vi "Picture_shr_Save_to_matlab.vi"(8 "Input Cluster":T7, 9 "Stack":T1, 10 "Mode":enum32{"Confocal", "High Res"}(radio), 11 "Save":bool) -> ()   [LabVIEW 2009]
uses:
  atmcd32d.llb/AcquisitionMode_mode typedef.ctl
  atmcd32d.llb/ReadMode_mode typedef.ctl
  atmcd32d.llb/TriggerMode_mode typedef.ctl
  atmcd32d.llb/Shutter_type typedef.ctl
  atmcd32d.llb/Shutter_mode typedef.ctl
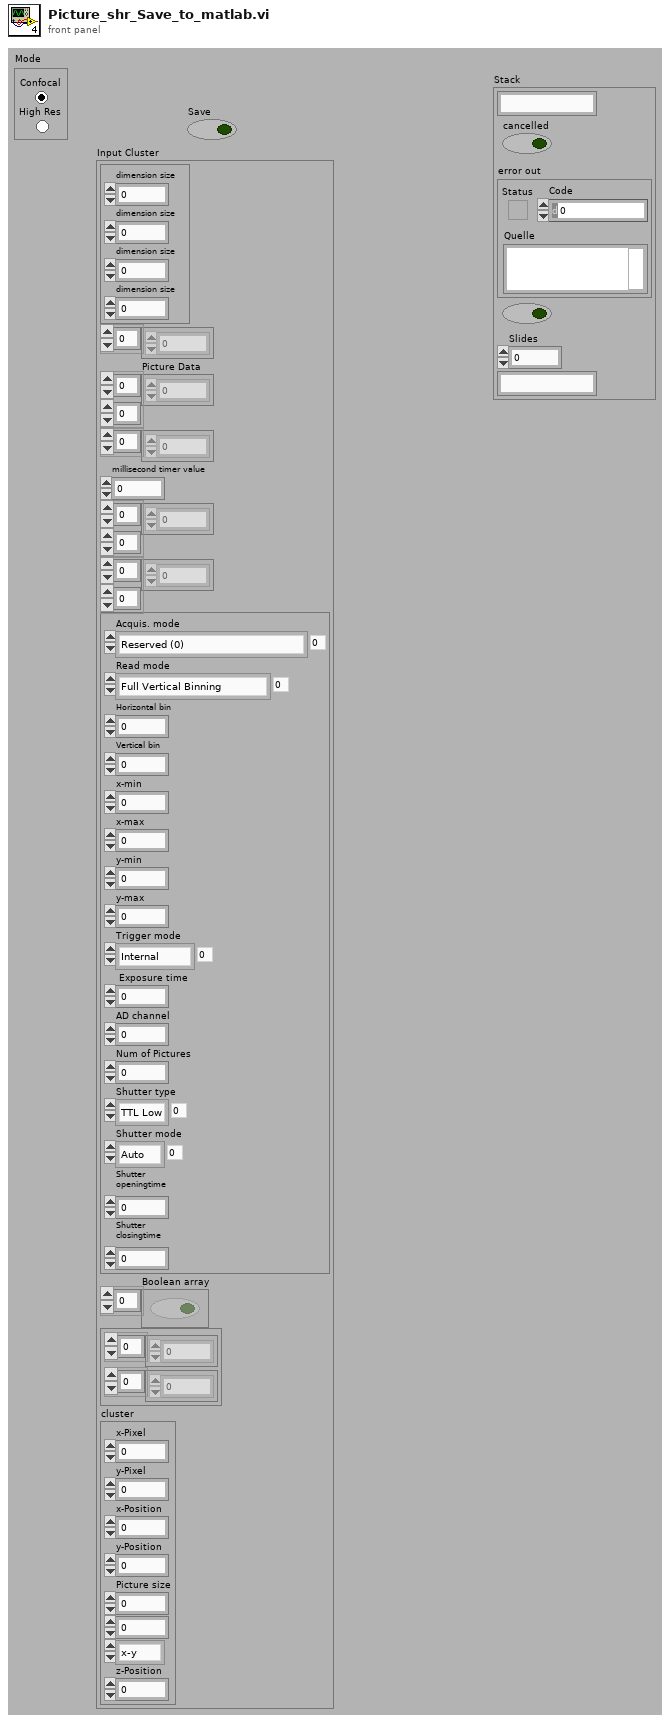
[diagram p1: front panel]
types:
  T1 = cluster{string, "cancelled":bool, "error out":errorcluster, bool, "Slides":i32, string}
  T2 = typedef "AcquisitionMode_mode typedef.ctl" = enum16{"Reserved (0)", "Single Scan", "Accumulate", "Kinetics", "Fast Kinetics", "Run Till Abort", "Reserved (6)", "Reserved (7)", "Reserved (8)", "Time Delayed Integration"}
  T3 = typedef "ReadMode_mode typedef.ctl" = enum16{"Full Vertical Binning", "Multi-Track", "Random-Track", "Single-Track", "Image"}
  T4 = typedef "TriggerMode_mode typedef.ctl" = enum16{"Internal", "External", "N/A (2)", "N/A (3)", "N/A (4)", "N/A (5)", "External Start"}
  T5 = typedef "Shutter_type typedef.ctl" = enum16{"TTL Low", "TTL High"}
  T6 = typedef "Shutter_mode typedef.ctl" = enum16{"Auto", "Open", "Close"}
  T7 = cluster{cluster{"dimension size":i32, "dimension size":i32, "dimension size":i32, "dimension size":i32}, i32[], "Picture Data":dbl[][], u32[], "millisecond timer value":u32, dbl[][], i32[][], cluster{"Acquis. mode":T2, "Read mode":T3, "Horizontal bin":i32, "Vertical bin":i32, "x-min":i32, "x-max":i32, "y-min":i32, "y-max":i32, "Trigger mode":T4, " Exposure time":sgl, "AD channel":i32, "Num of Pictures":i32, "Shutter type":T5, "Shutter mode":T6, "Shutter\nopeningtime":i32, "Shutter\nclosingtime":i32}, "Boolean array":bool[], cluster{dbl[], dbl[]}, "cluster":cluster{"x-Pixel":u16, "y-Pixel":u16, "x-Position":dbl, "y-Position":dbl, "Picture size":dbl, dbl, enum32{"x-y", "x-z", "y-z"}, "z-Position":dbl}}
  T8 = enum16{"open", "replace", "create", "open or create", "replace or create", "replace or create with confirmation"}
  T9 = cluster{"x-Pixel":u16, "y-Pixel":u16, "x-Position":dbl, "y-Position":dbl, "Picture size":dbl, dbl, enum32{"x-y", "x-z", "y-z"}, "z-Position":dbl}
  T10 = cluster{"Acquis. mode":T2, "Read mode":T3, "Horizontal bin":i32, "Vertical bin":i32, "x-min":i32, "x-max":i32, "y-min":i32, "y-max":i32, "Trigger mode":T4, " Exposure time":sgl, "AD channel":i32, "Num of Pictures":i32, "Shutter type":T5, "Shutter mode":T6, "Shutter\nopeningtime":i32, "Shutter\nclosingtime":i32}
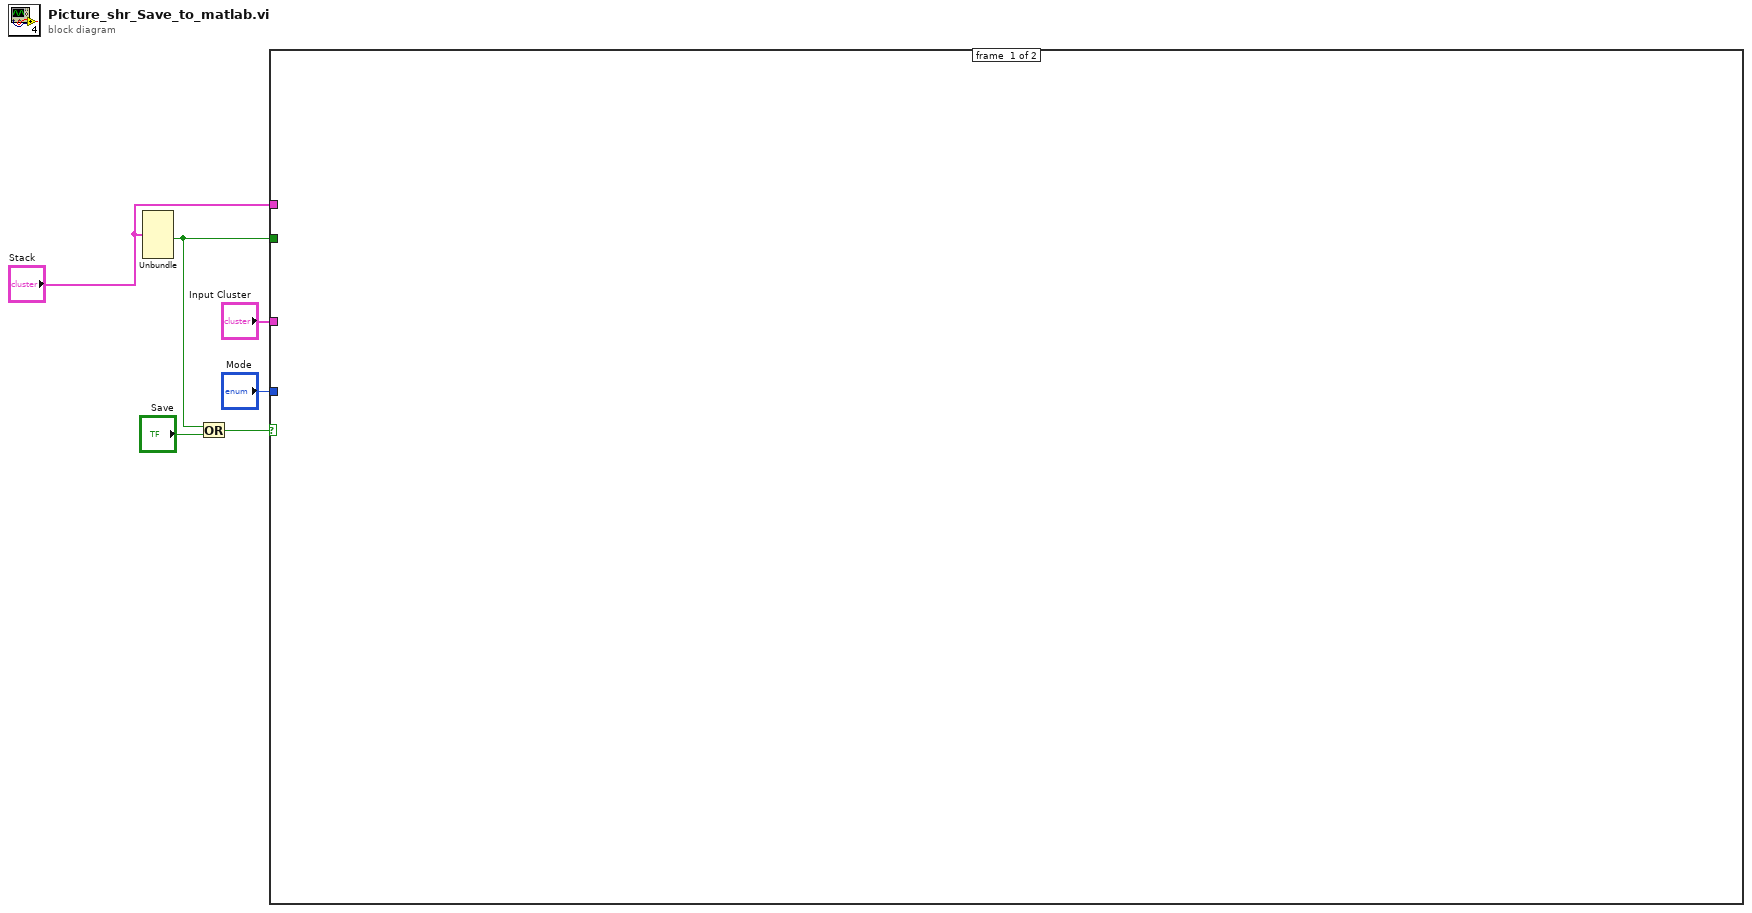
[diagram p0: block diagram]
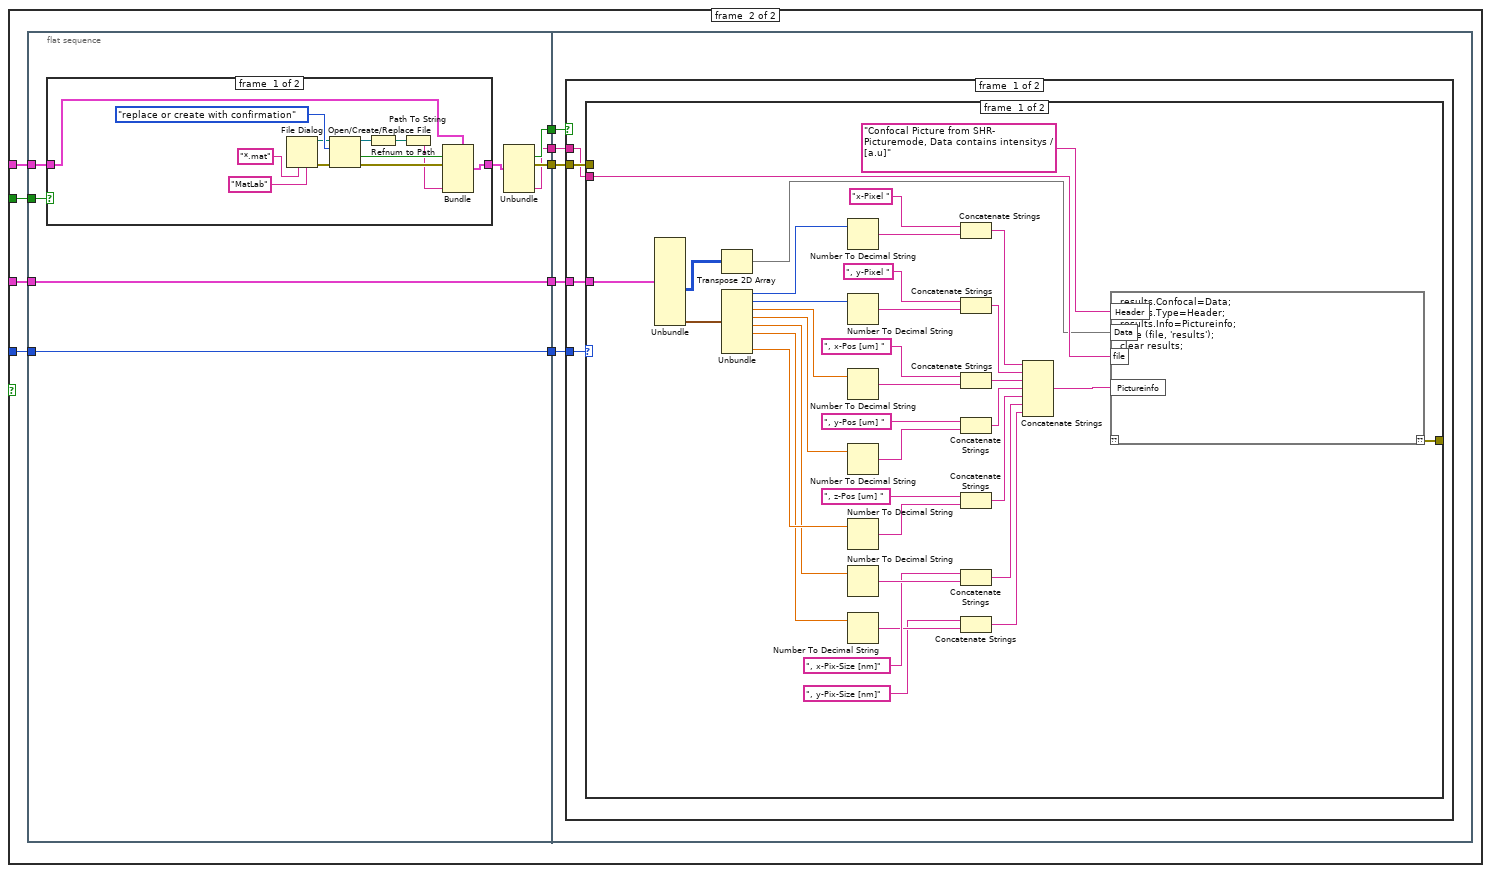
[diagram p2: hidden frame]
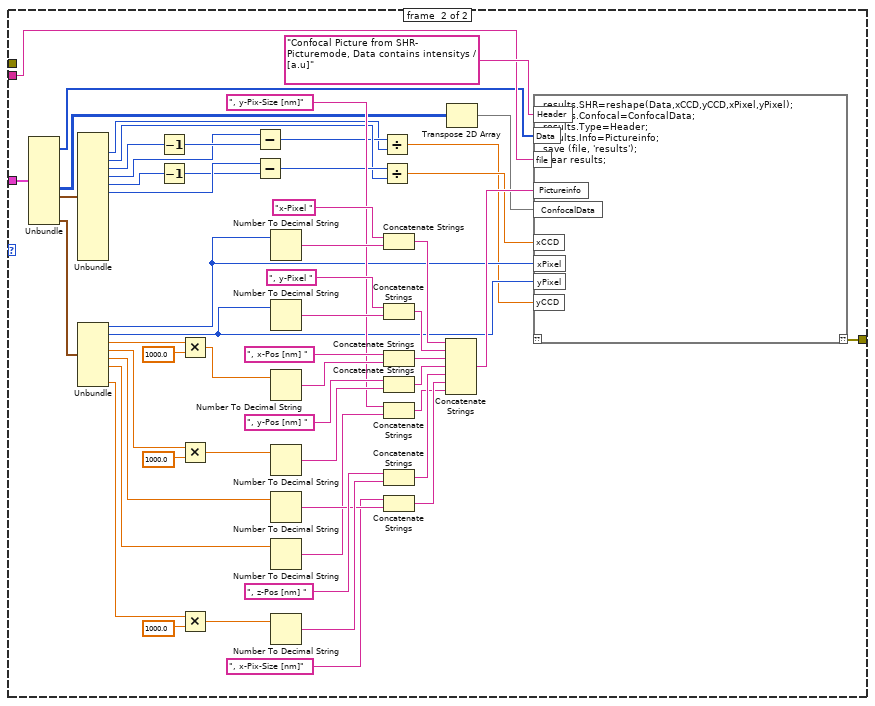
[diagram p4: hidden frame]
diagram:
  n1 = Unbundle("Stack") -> (w4:bool)  [unwired: 5 out]
  n2 = Or(x=w4, y="Save") -> (x .or. y?=w2:bool)
  n3 = case shown="True" w2 {
    tunnel: "Mode" -> [_ w15]
    tunnel: "Input Cluster" -> [_ w10]
    tunnel: "Stack" -> [_ w8]
    tunnel: w4 -> [_ w7]
    frame #0 {
    }
    frame #1 {
      n4 = flat-sequence {
        tunnel: w15 -> [w23]
        tunnel: [w23] -> w14
        tunnel: [w19] -> w13
        tunnel: [w20] -> w12
        tunnel: [w22] -> w11
        tunnel: w10 -> [w22]
        tunnel: [w16] -> w9
        tunnel: w8 -> [w18]
        tunnel: w7 -> [w17]
        tunnel: w14 -> [w41]
        tunnel: w13 -> [w39]
        tunnel: w12 -> [w40]
        tunnel: w11 -> [w37]
        tunnel: w9 -> [w38]
        frame #0 {
          n5 = case shown="False" w17 {
            tunnel: [w28 w36] -> w21
            tunnel: w18 -> [w25 w36]
            frame #0 {
              n6 = File Dialog(4:"MatLab" ("pattern label"), 6:"*.mat" ("pattern (all files)")) -> (0:w33:errorcluster, 3:w34:path)  [unwired: 1 in, 6 out]
              n7 = Open/Create/Replace File(file path (use dialog)=w34, error in=w33, operation (0:open)=T8."replace or create with confirmation") -> (refnum out=w30:refnum<file>, cancelled=w26:bool, error out=w27:errorcluster)  [unwired: 3 out]
              n8 = Refnum to Path(1:w30) -> (0:w29:path)
              n9 = Path To String(path=w29) -> (string=w24:string)
              n10 = Bundle(cluster=w25, "cancelled"=w26, "error out"=w27, w24) -> (w28:T1)  [unwired: 3 out]
            }
            frame #1 {
            }
          }
          n11 = Unbundle(w21) -> ("cancelled"=w19:bool, "error out"=w20:errorcluster, w16:string)  [unwired: 3 out]
        }
        frame #1 {
          n12 = case shown="False" w39 {
            tunnel: w41 -> [w45 _]
            tunnel: w40 -> [w44 _]
            tunnel: w38 -> [w43 _]
            tunnel: w37 -> [w42 _]
            frame #0 {
              n13 = case shown="\"High Res\"" w45 {
                tunnel: w44 -> [_ _]
                tunnel: w43 -> [w79 w110]
                tunnel: w42 -> [w80 w111]
                tunnel: [w46 w91] -> _
                frame #0 {
                  n14 = Unbundle(w80) -> (w48:i32[][], "cluster"=w78:T9)  [unwired: 9 out]
                  n15 = Transpose 2D Array(2D array=w48) -> (transposed array=w47:i32[][])
                  n16 = Unbundle(w78) -> ("x-Pixel"=w77:u16, "y-Pixel"=w71:u16, "x-Position"=w67:dbl, "y-Position"=w63:dbl, "Picture size"=w55:dbl, w51:dbl, "z-Position"=w59:dbl)  [unwired: 1 out]
                  n17 = Number To Decimal String(number=w77) -> (decimal integer string=w76:string)  [unwired: 1 out]
                  n18 = Number To Decimal String(number=w71) -> (decimal integer string=w73:string)  [unwired: 1 out]
                  n19 = Number To Decimal String(number=w67) -> (decimal integer string=w69:string)  [unwired: 1 out]
                  n20 = Number To Decimal String(number=w63) -> (decimal integer string=w65:string)  [unwired: 1 out]
                  n21 = Number To Decimal String(number=w59) -> (decimal integer string=w61:string)  [unwired: 1 out]
                  n22 = Number To Decimal String(number=w55) -> (decimal integer string=w57:string)  [unwired: 1 out]
                  n23 = Number To Decimal String(number=w51) -> (decimal integer string=w53:string)  [unwired: 1 out]
                  n24 = Concatenate Strings("x-Pixel " ("String"), w76) -> (w74:string)
                  n25 = Concatenate Strings(", y-Pixel " ("String"), w73) -> (w70:string)
                  n26 = Concatenate Strings(", x-Pos [um] " ("String"), w69) -> (w66:string)
                  n27 = Concatenate Strings(", y-Pos [um] " ("String"), w65) -> (w62:string)
                  n28 = Concatenate Strings(", z-Pos [um] " ("String"), w61) -> (w58:string)
                  n29 = Concatenate Strings(", x-Pix-Size [nm]" ("String"), w57) -> (w54:string)
                  n30 = Concatenate Strings(", y-Pix-Size [nm]" ("String"), w53) -> (w50:string)
                  n31 = Concatenate Strings(w74, w70, w66, w62, w58, w54, w50) -> (w49:string)
                  n32 = script code="results.Confocal=Data;\nresults.Type=Header;\nresults.Info=Pictureinfo;\nsave (file, 'results');\nclear results;"("file"=w79, "Data"=w47, "Header"="Confocal Picture from SHR- Picturemode, Data contains intensitys / [a.u]" ("String"), "Pictureinfo"=w49) -> ("??"=w46:errorcluster)  [unwired: 1 out]
                }
                frame #1 {
                  n33 = Unbundle(w111) -> (w98:i32[], w100:i32[][], w107:T10, "cluster"=w136:T9)  [unwired: 7 out]
                  n34 = Unbundle(w107) -> ("Horizontal bin"=w92:i32, "Vertical bin"=w102:i32, "x-min"=w94:i32, "x-max"=w93:i32, "y-min"=w106:i32, "y-max"=w105:i32)  [unwired: 10 out]
                  n35 = Unbundle(w136) -> ("x-Pixel"=w109:u16, "y-Pixel"=w108:u16, "x-Position"=w89:dbl, "y-Position"=w86:dbl, "Picture size"=w118:dbl, w114:dbl, "z-Position"=w83:dbl)  [unwired: 1 out]
                  n36 = Decrement(x=w94) -> (x-1=w97:i32)
                  n37 = Decrement(x=w106) -> (x-1=w104:i32)
                  n38 = Multiply(x=w89, y=1000.0) -> (x*y=w88:dbl)
                  n39 = Multiply(x=w86, y=1000.0) -> (x*y=w85:dbl)
                  n40 = Multiply(x=w83, y=1000.0) -> (x*y=w82:dbl)
                  n41 = Subtract(x=w93, y=w97) -> (x-y=w96:i32)
                  n42 = Subtract(x=w105, y=w104) -> (x-y=w103:i32)
                  n43 = Number To Decimal String(number=w109) -> (decimal integer string=w135:string)  [unwired: 1 out]
                  n44 = Number To Decimal String(number=w108) -> (decimal integer string=w132:string)  [unwired: 1 out]
                  n45 = Number To Decimal String(number=w88) -> (decimal integer string=w129:string)  [unwired: 1 out]
                  n46 = Number To Decimal String(number=w85) -> (decimal integer string=w126:string)  [unwired: 1 out]
                  n47 = Number To Decimal String(number=w118) -> (decimal integer string=w120:string)  [unwired: 1 out]
                  n48 = Number To Decimal String(number=w114) -> (decimal integer string=w116:string)  [unwired: 1 out]
                  n49 = Number To Decimal String(number=w82) -> (decimal integer string=w123:string)  [unwired: 1 out]
                  n50 = Divide(x=w96, y=w92) -> (x/y=w95:dbl)
                  n51 = Divide(x=w103, y=w102) -> (x/y=w101:dbl)
                  n52 = Concatenate Strings("x-Pixel " ("String"), w135) -> (w133:string)
                  n53 = Concatenate Strings(", y-Pixel " ("String"), w132) -> (w130:string)
                  n54 = Concatenate Strings(", x-Pos [nm] " ("String"), w129) -> (w127:string)
                  n55 = Concatenate Strings(", y-Pos [nm] " ("String"), w126) -> (w124:string)
                  n56 = Concatenate Strings(", y-Pix-Size [nm]" ("String"), w116) -> (w113:string)
                  n57 = Concatenate Strings(", z-Pos [nm] " ("String"), w123) -> (w121:string)
                  n58 = Concatenate Strings(", x-Pix-Size [nm]" ("String"), w120) -> (w117:string)
                  n59 = Concatenate Strings(w133, w130, w127, w124, w121, w117, w113) -> (w112:string)
                  n60 = Transpose 2D Array(2D array=w100) -> (transposed array=w99:i32[][])
                  n61 = script code="results.SHR=reshape(Data,xCCD,yCCD,xPixel,yPixel);\nresults.Confocal=ConfocalData;\nresults.Type=Header;\nresults.Info=Pictureinfo;\nsave (file, 'results');\nclear results;"("file"=w110, "Data"=w98, "Header"="Confocal Picture from SHR- Picturemode, Data contains intensitys / [a.u]" ("String"), "Pictureinfo"=w112, "xCCD"=w101, "xPixel"=w109, "yPixel"=w108, "ConfocalData"=w99, "yCCD"=w95) -> ("??"=w91:errorcluster)  [unwired: 1 out]
                }
              }
            }
            frame #1 {
            }
          }
        }
      }
    }
  }
